vi "FindIndexByID.vi"(8 "error in (no error)":errorcluster, 10 "id":string, 11 "registry":T1[](array[typedef])) -> (0 "error out":errorcluster, 2 "index":i32, 3 "found":bool, 5 "registryEntry":T1)   [LabVIEW 2026, in "Lumberjack.lvlib" / "LogManager.lvclass"]
uses:
  LogManager.lvclass
  TypeDefs/RegistryEntry.ctl
  <vilib>/ActorFramework/Message Enqueuer/Message Enqueuer.lvclass
  LogManager.lvclass/LogManager.ctl
  Lumberjack.lvlib
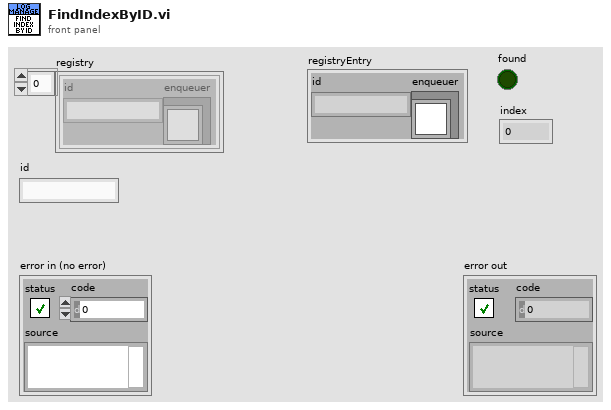
[diagram p1: front panel]
types:
  T1 = typedef "Lumberjack.lvlib/RegistryEntry.ctl" = cluster{"id":string, "enqueuer":refnum<class "Message Enqueuer.lvclass">}
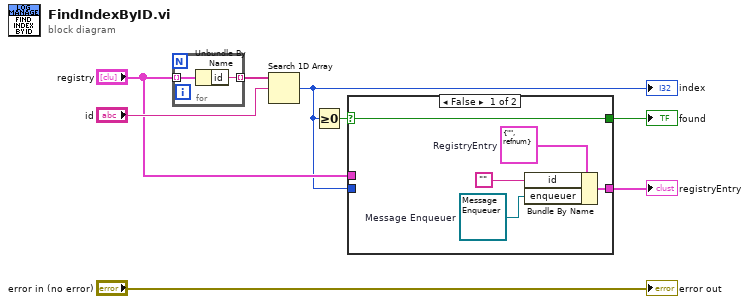
[diagram p0: block diagram]
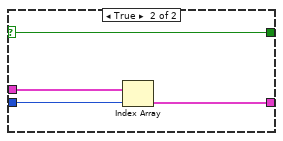
[diagram p2: hidden frame]
diagram:
  n1 = for {
    tunnel: "registry" -> [w10] mode=indexing
    tunnel: [w9] -> w8 mode=indexing
    n2 = Unbundle By Name(w10) -> ("id"=w9:string)
  }
  n3 = Search 1D Array(1D array=w8, element="id") -> (index of element=w4:i32)  [unwired: 1 in]
  "index" <- w4
  n4 = Greater Or Equal To 0?(x=w4) -> (x >= 0?=w3:bool)
  n5 = case shown="False" w3 {
    selector: w3 -> [w11 w17]
    tunnel: "registry" -> [_ w19]
    tunnel: w4 -> [_ w18]
    tunnel: [w11 w17] -> w2
    tunnel: [w12 w16] -> w1
    frame False {
      w15 = T1 {"id"="", "enqueuer"=refnum}  # RegistryEntry
      w13 = refnum<class "Message Enqueuer.lvclass"> refnum  # Message Enqueuer
      n6 = Bundle By Name(cluster=w15, "id"="", "enqueuer"=w13) -> (w12:T1)
    }
    frame True {
      n7 = Index Array(array=w19, index=w18) -> (element=w16:T1)
    }
  }
  "found" <- w2
  "registryEntry" <- w1
  "error out" <- "error in (no error)"
